vi "Apply.vi"(8 "error in":errorcluster, 11 "AI Voltage DAQmx Cont CFG in":refnum<class "AI Voltage DAQmx Cont CFG Simulated.lvclass">) -> (0 "error out":errorcluster, 3 "AI Voltage DAQmx Cont CFG out":refnum<class "AI Voltage DAQmx Cont CFG Simulated.lvclass">)   [LabVIEW 2024, in "DAQmx Simulated CFGs.lvlib" / "AI Voltage DAQmx Cont CFG Simulated.lvclass"]
uses:
  AI Voltage DAQmx Cont CFG Simulated.lvclass
  Configurations/CFG Base/CFG Base.lvclass/CFG Base.ctl
  AI Voltage DAQmx Cont CFG/AI Voltage DAQmx Cont CFG.lvclass
  Configurations/CFG Base/CFG Base.lvclass
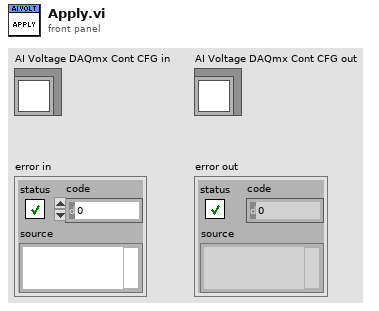
[diagram p1: front panel]
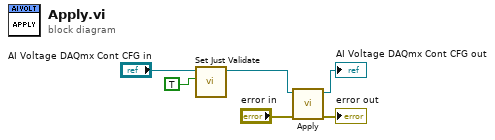
[diagram p0: block diagram]
diagram:
  n1 = call "Set Just Validate.vi"("Just Validate"=TRUE, "CFG Base in"="AI Voltage DAQmx Cont CFG in") -> ("CFG Base out"=w2:refnum<class "AI Voltage DAQmx Cont CFG Simulated.lvclass">)  [unwired: 9 in]
  n2 = call-parent "Apply.vi"("error in"="error in", "DAQmx Base CFG in"=w2) -> ("error out"=→"error out":errorcluster, "DAQmx Base CFG out"=→"AI Voltage DAQmx Cont CFG out":refnum<class "AI Voltage DAQmx Cont CFG Simulated.lvclass">)  [unwired: 8 in]
